vi "Error-For.vi"() -> ()   [LabVIEW 2020]
panel:
  out "Numeric":i32
  in  "stop":bool
  out "error out":errorcluster
  in  "error in":errorcluster
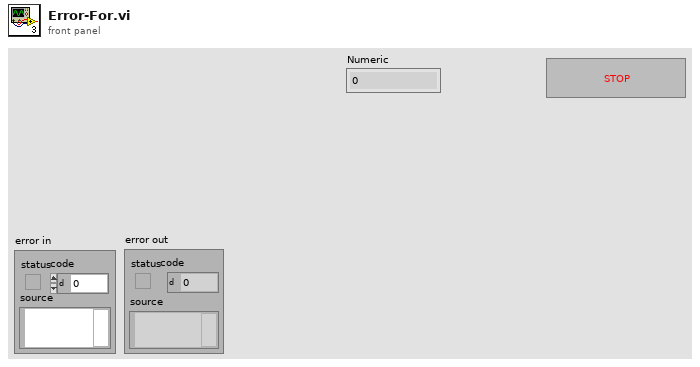
[diagram p1: front panel]
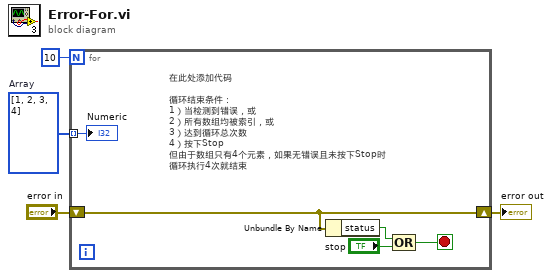
[diagram p0: block diagram]
diagram:
  w1 = i32[] [1, 2, 3, 4]  # Array
  n1 = for {
    N: 10 -> [_]
    shift-right: [w6] -> w2
    shift-left: "error in" -> [w6]
    tunnel: w1 -> [w5] mode=indexing
    stop <- w7 stop-if-true
    # "在此处添加代码\n\n循环结束条件：\n1）当检测到错误，或\n2）所有数组均被索引，或\n3）达到循环总次数\n4）按下Stop\n但由于数组只有4个元素，如果无错误且未按下Stop时\n循环执行4次就结束"
    n2 = Unbundle By Name(w6) -> ("status"=w8:bool)
    n3 = Compound Arithmetic op=OR(w8, "stop") -> (w7:bool)
    "Numeric" <- w5
  }
  "error out" <- w2
